vi "Untitled 1.vi"() -> ()   [LabVIEW 2020]
panel:
  out "length":i32
  out "Boolean":bool
  out "String 4":string
  in  "stop":bool
  out "String 2":string="case1"
  out "String":string="case 1"
  in  "case":dbl
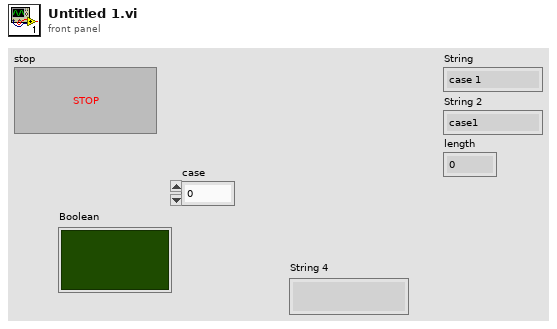
[diagram p1: front panel]
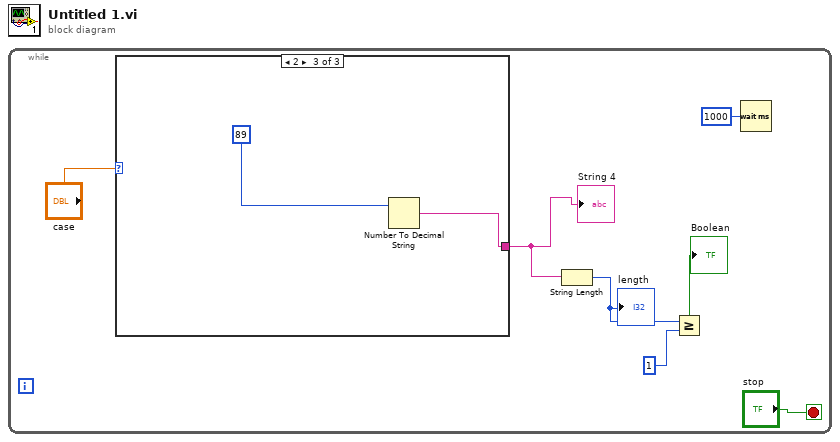
[diagram p0: block diagram]
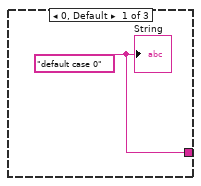
[diagram p2: hidden frame]
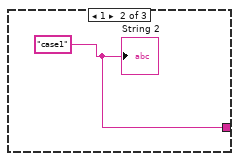
[diagram p3: hidden frame]
diagram:
  n1 = while {
    stop <- "stop" stop-if-true
    n2 = case shown="2" "case" {
      tunnel: [w8 w9 w10] -> w4
      frame 0, Default {
        w8 = "default case 0"
        "String" <- w8
      }
      frame 1 {
        w9 = "case1"
        "String 2" <- w9
      }
      frame 2 {
        n3 = Number To Decimal String(number=89) -> (decimal integer string=w10:string)  [unwired: 1 in]
      }
    }
    "String 4" <- w4
    n4 = String Length(string=w4) -> (length=w3:i32)
    "length" <- w3
    n5 = Greater Or Equal?(x=w3, y=1) -> (x >= y?=→"Boolean":bool)
    n6 = Wait (ms)(milliseconds to wait=u32 1000) -> ()  [unwired: 1 out]
  }
